vi "pb-program.vi"(10 "Commands":T1(array[cluster]) {"Time" format="%.3p"; "Op Code" items=["Continue", "Stop", "Loop", "End Loop", "JSR", "RTS", "Branch", "Long Delay", "Wait"]}) -> (3 "path out":path)   [LabVIEW 2018]
uses:
  GLOBAL_VAR.vi
panel:
  # "1"
  # "2"
  # "3"
  # "4"
  # "5"
  # "6"
  # "7"
  # "8"
  # "9"
  # "10"
  # "11"
  # "12"
  # "13"
  # "14"
  # "15"
  # "16"
  # "17"
  # "18"
  # "19"
  # "20"
  # "21"
  # "22"
  # "23"
  # "24"
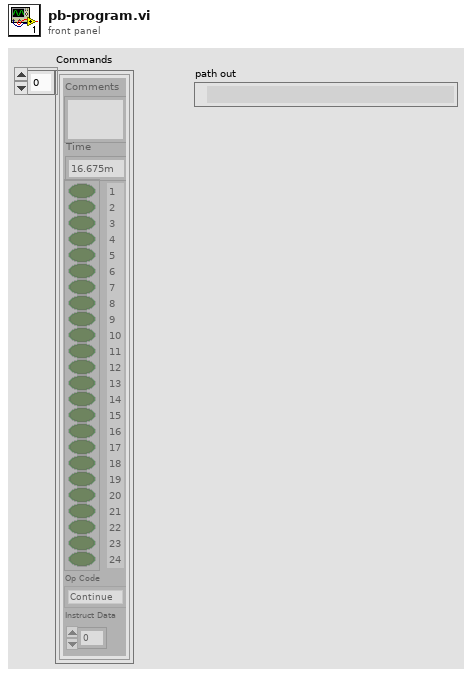
[diagram p1: front panel]
types:
  T1 = cluster{"Instruct Data":i32, "Op Code":i32, "Flags":bool[], "Comments":string, "Time":dbl}[]
  T2 = enum16{"Pulse Program", "Frequency Registers", "TX Phase Registers", "RX Phase Registers"}
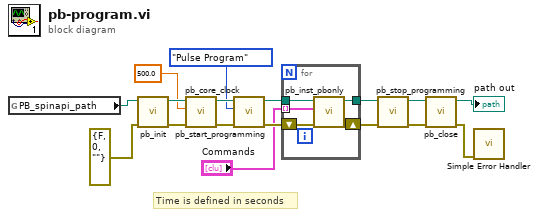
[diagram p0: block diagram]
diagram:
  # "Time is defined in seconds"
  n1 = global read "GLOBAL_VAR.vi" "PB_spinapi_path"() -> (w1:path)
  n2 = call "pb_init.vi"("error in (no error)"=errorcluster {"status"=FALSE, "code"=0, "source"=""} ("error constant"), "path in"=w1) -> ("error out"=w16:errorcluster, "path out"=w17:path)  [unwired: 8 in]
  n3 = call "pb_core_clock.vi"("error in (no error)"=w16, "clock_freq (MHz)"=500.0, "path in"=w17) -> ("error out"=w13:errorcluster, "path out"=w14:path)  [unwired: 7 in]
  n4 = call "pb_start_programming.vi"("error in (no error)"=w13, "Device"=T2."Pulse Program", "path in"=w14) -> ("error out"=w8:errorcluster, "path out"=w9:path)  [unwired: 7 in]
  n5 = for {
    tunnel: "Commands" -> [w22] mode=indexing
    tunnel: [w21] -> w7
    tunnel: w9 -> [w20]
    shift-right: [w18] -> w6
    shift-left: w8 -> [w19]
    n6 = call "pb_inst_pbonly.vi"("error in (no error)"=w19, "PB Instruction"=w22, "path in"=w20) -> ("error out"=w18:errorcluster, "path out"=w21:path)  [unwired: 7 in]
  }
  n7 = call "pb_stop_programming.vi"("error in (no error)"=w6, "path in"=w7) -> ("error out"=w10:errorcluster, "path out"=w11:path)  [unwired: 8 in]
  n8 = call "pb_close.vi"("error in (no error)"=w10, "path in"=w11) -> ("error out"=w2:errorcluster, "path out"=→"path out":path)  [unwired: 8 in]
  n9 = call <vilib>:"Simple Error Handler.vi"("error in (no error)"=w2) -> ()  [unwired: 4 in, 5 out]
